vi "UPINFO.vi"(0 "总成追溯码":string, 1 "工位追溯码":string, 2 "产品型号":string, 3 "设备编号":string, 4 "操作员":string, 5 "error in (no error)":errorcluster caption="错误输入（无错误）", 6 "加工状态":string) -> (19 "error out":errorcluster caption="错误输出")   [LabVIEW 2019]
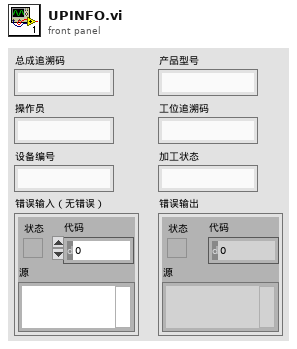
[diagram p1: front panel]
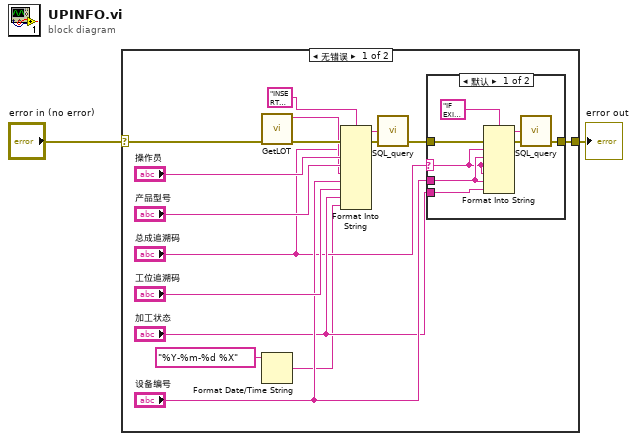
[diagram p0: block diagram]
diagram:
  n1 = case shown="无错误" "error in (no error)" {
    selector: "error in (no error)" -> [w13 w28]
    tunnel: [w7 w28] -> w1
    frame No Error {
      n2 = call "GetLOT.vi"("错误输入"=w13) -> ("错误输出"=w12:errorcluster, "LOT"=w11:string)  [unwired: 8 in, 1 out]
      n3 = Format Date/Time String(time format string (%c)="%Y-%m-%d %X" ("时间格式字符串(%c)")) -> (date/time string=w3:string)  [unwired: 2 in]
      n4 = Format Into String(format string="INSERT INTO [SanliServer].[dbo].[产品质量1] (\n\t[总成追溯码],\n\t[操作员],\n\t[产品型号],\n\t[生产编号],\n\t[设备编号],\n\t[工位追溯码],\n\t[加工状态],\n [时间]\n)VALUES\n\t(\n\t\tN'%s',\n\t\tN'%s',\n\t\tN'%s',\n\t\tN'%s',\n\t\tN'%s',\n\t\tN'%s',\n\t\tN'%s',\n  N'%s'\n\t)", error in=w12, "总成追溯码", "操作员", "产品型号", w11, "设备编号", "工位追溯码", "加工状态", w3) -> (resulting string=w15:string, error out=w14:errorcluster)  [unwired: 1 in]
      n5 = call "SQL_query.vi"("error in (no error)"=w14, "SQL query"=w15) -> ("error out"=w8:errorcluster)  [unwired: 1 in, 2 out]
      n6 = case shown="默认" "总成追溯码" {
        selector: "总成追溯码" -> [w20 _]
        tunnel: "设备编号" -> [w26 _]
        tunnel: "加工状态" -> [w25 _]
        tunnel: w8 -> [w24 w27]
        tunnel: [w22 w27] -> w7
        frame Default {
          n7 = Format Into String(format string="IF EXISTS (\n\tSELECT\n\t\t*\n\tFROM\n\t\t[生产状态]\n\tWHERE\n\t\t[总成追溯码] = '%s'\n) UPDATE [生产状态]\nSET [最后加工工位] = '%s'\nWHERE\n\t[总成追溯码] = '%s'\nELSE\n\tINSERT INTO [生产状态] (\n\t\t[总成追溯码],\n\t\t[最后加工工位],\n\t\t[工件状态]\n\t)\nVALUES\n\t('%s', '%s', '%s')", error in=w24, w20, w26, w20, w20, w26, w25) -> (resulting string=w21:string, error out=w23:errorcluster)  [unwired: 1 in]
          n8 = call "SQL_query.vi"("error in (no error)"=w23, "SQL query"=w21) -> ("error out"=w22:errorcluster)  [unwired: 1 in, 2 out]
        }
        frame "" {
        }
      }
    }
    frame Error {
    }
  }
  "error out" <- w1
